vi "Load DSF Configuration File.vi"(8 "error in (no error)":errorcluster, 10 "Path":path, 11 "Application Refs":T1) -> (0 "error out":errorcluster, 3 "Application Data out":T1)   [LabVIEW 2017, in "DSF Configuration Utility.lvlib"]
uses:
  DSF Configuration Utility.lvlib
  Application Data.ctl
  DSF Configuration API/1.0.0/Public/Controls/DSF Config Data RefNum.ctl
  Window State.ctl
  View Mode.ctl
  DSF Configuration API/1.0.0/DSF Configuration API.lvlib
panel:
  # "App\nData"
  # "App\nData"
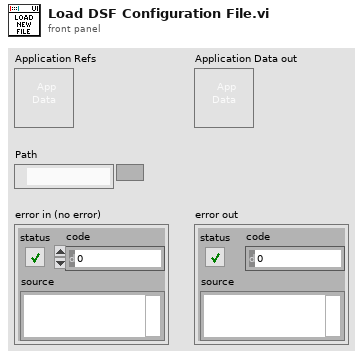
[diagram p1: front panel]
types:
  T1 = typedef "DSF Configuration Utility.lvlib/Application Data.ctl" = cluster{"DSF Refnum out":T2, "Tree Control":refnum<vi>, "Tab Control":refnum<vi>, "Top-Level VI":refnum<vi>, "value control refs":refnum<vi>[], "View State":T3}
  T2 = typedef "DSF Configuration API.lvlib/DSF Config Data RefNum.ctl" = refnum<k1>
  T3 = typedef "DSF Configuration Utility.lvlib/View Mode.ctl" = enum16{"Tree", "List"}
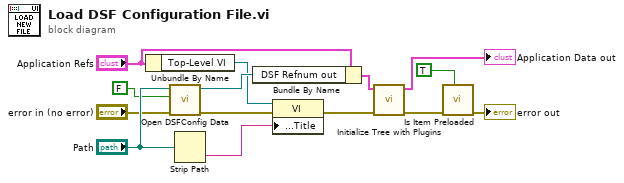
[diagram p0: block diagram]
diagram:
  n1 = Unbundle By Name("Application Refs") -> ("Top-Level VI"=w4:refnum<vi>)
  n2 = call "Open DSFConfig Data.vi"("error in (no error)"="error in (no error)", "create file if necessary (T)"=FALSE, "configuration file path"="Path") -> ("error out"=w13:errorcluster, "refnum"=w8:T2)  [unwired: 5 in, 2 out]
  n3 = Strip Path(path="Path") -> (name=w12:string)  [unwired: 1 out]
  n4 = Bundle By Name(cluster="Application Refs", "DSF Refnum out"=w8) -> (w7:T1)
  n5 = property class="VI"(reference=w4, error in=w13, "Front Panel.Title"=w12) -> (error out=w14:errorcluster)  [unwired: 1 out]
  n6 = call "Initialize Tree with Plugins.vi"("error in (no error)"=w14, "Application Data in"=w7) -> ("error out"=w3:errorcluster, "Application Data out"=→"Application Data out":T1)  [unwired: 8 in]
  n7 = call "Is Item Preloaded"("clear entries"=TRUE, "error in (no error)"=w3) -> ("error out"=→"error out":errorcluster)  [unwired: 7 in, 2 out]
